vi "RoiLoopAndorEins.vi"(8 "error in":errorcluster, 11 "queue in":refnum<queue>) -> (0 "error out":errorcluster, 3 "Intensity Graph Andor One":i32[][](graph))   [LabVIEW 2011]
panel:
  out "queue out":refnum<queue>
  in  "OldDatain":i32[][](array[numeric])
  in  "Array":i32[][][](array[numeric])
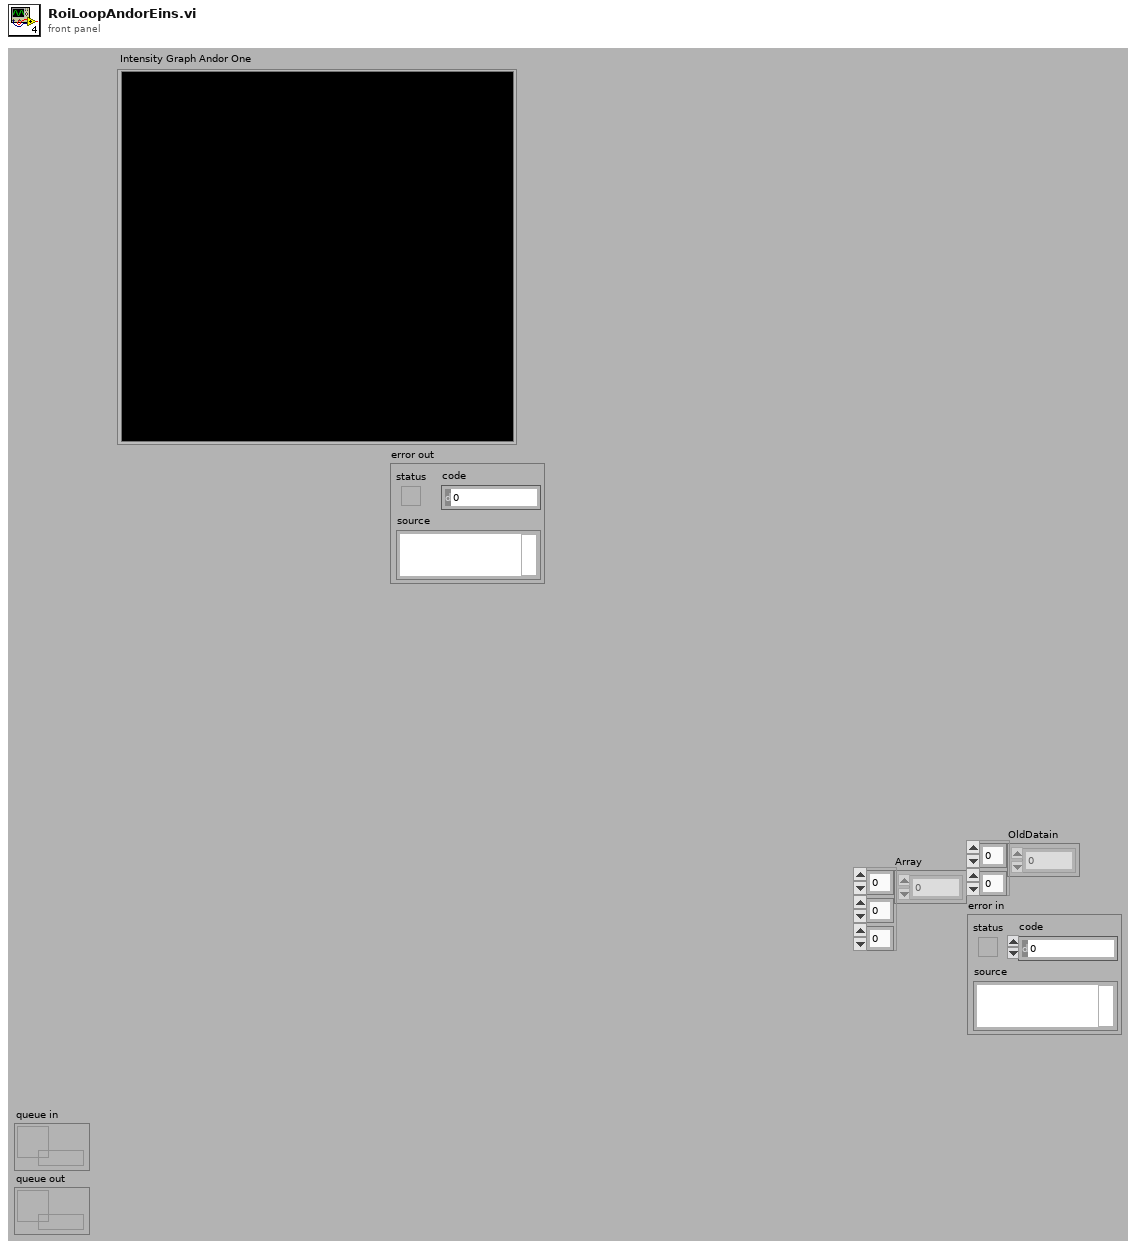
[diagram p1: front panel]
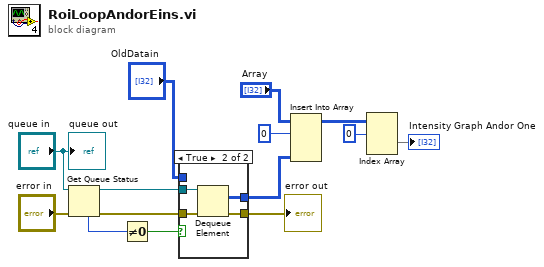
[diagram p0: block diagram]
diagram:
  n1 = Get Queue Status(queue="queue in", error in (no error)="error in") -> (queue out=w13:refnum<queue>, error out=w11:errorcluster, # elements in queue=w10:i32)  [unwired: 1 in, 5 out]
  n2 = Not Equal To 0?(x=w10) -> (x != 0?=w12:bool)
  n3 = case shown="True" w12 {
    tunnel: w11 -> [w16 w20]
    tunnel: [w16 w18] -> w1
    tunnel: w13 -> [_ w19]
    tunnel: [w15 w17] -> w5
    tunnel: "OldDatain" -> [w15 _]
    frame False {
    }
    frame True {
      n4 = Dequeue Element(queue=w19, error in (no error)=w20) -> (element=w17:i32[][], error out=w18:errorcluster)  [unwired: 1 in, 2 out]
    }
  }
  "error out" <- w1
  n5 = Insert Into Array(array="Array", index (dim 0)=0 ("index (page)"), new element=w5) -> (w8:i32[][][])  [unwired: 2 in]
  n6 = Index Array(array=w8, index (dim 0)=0 ("index (page)")) -> (element=→"Intensity Graph Andor One":i32[][])  [unwired: 2 in]
  "queue out" <- "queue in"
